vi "Remove Type Specialization Structure.vi"(8 "error in (no error)":errorcluster, 11 "VI Ref In":refnum<vi>) -> (0 "error out":errorcluster, 3 "VI Ref Out":refnum<vi>)   [LabVIEW 2020]
doc: "Removes the Type Specialization structure from the VI. The active case is first shown, then the structure removed to retain the correctly executable code."
uses:
  <vilib>/Utility/traverseref.llb/TRef TravTarget.ctl
  <vilib>/Utility/traverseref.llb/VI Scripting - Traverse.lvlib
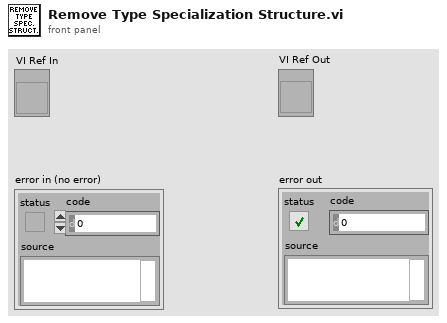
[diagram p1: front panel]
types:
  T1 = typedef "TRef TravTarget.ctl" = enum16{"FP", "BD", "Other"}
  T2 = enum32{"Conditional Disable Style", "Diagram Disable Style", "Type Specialization Style"}
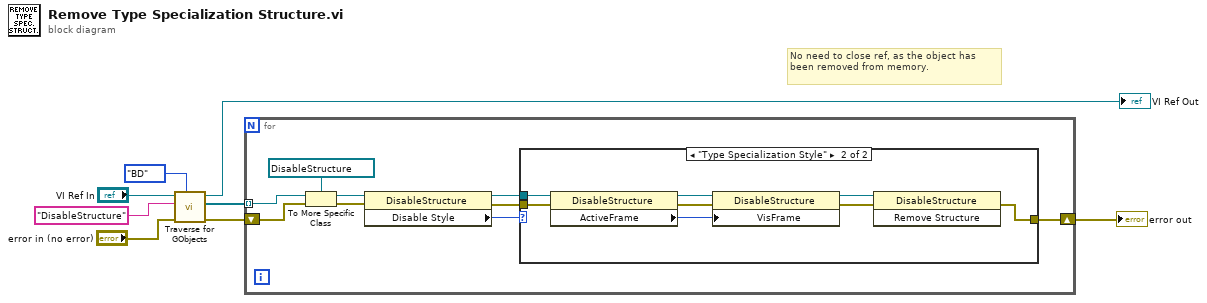
[diagram p0: block diagram]
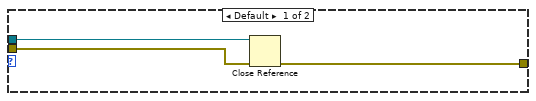
[diagram p2: hidden frame]
diagram:
  # "No need to close ref, as the object has been removed from memory."
  n1 = call <vilib>:"Traverse for GObjects.vi"("Traverse Target"=TRef_TravTarget."BD", "error in (no error)"="error in (no error)", "Class Name"="DisableStructure", "VI Refnum"="VI Ref In") -> ("error out"=w3:errorcluster, "References"=w5:refnum<vi>[], "dup VI Refnum"=→"VI Ref Out":refnum<vi>)  [unwired: 4 in, 1 out]
  n2 = for {
    tunnel: w5 -> [w16] mode=indexing
    shift-right: [w9] -> w2
    shift-left: w3 -> [w13]
    n3 = To More Specific Class(target class=refnum<vi> refnum ("reference"), reference=w16, error in=w13) -> (specific class reference=w15:refnum<vi>, error out=w12:errorcluster)
    n4 = property class="DisableStructure"(reference=w15, error in=w12) -> (reference out=w10:refnum<vi>, error out=w11:errorcluster, "Disable Style"=w14:T2)
    n5 = case shown="\"Type Specialization Style\"" w14 {
      tunnel: w11 -> [w19 w24]
      tunnel: w10 -> [w20 w25]
      tunnel: [w18 w21] -> w9
      frame Default {
        n6 = Close Reference(reference=w20, error in (no error)=w19) -> (error out=w18:errorcluster)
      }
      frame "Type Specialization Style" {
        n7 = property class="DisableStructure"(reference=w25, error in=w24) -> (reference out=w28:refnum<vi>, error out=w23:errorcluster, "ActiveFrame"=w27:i16)
        n8 = property class="DisableStructure"(reference=w28, error in=w23, "VisFrame"=w27) -> (reference out=w26:refnum<vi>, error out=w22:errorcluster)
        n9 = invoke class="DisableStructure" method="Remove Structure"(reference=w26, error in=w22) -> (error out=w21:errorcluster)  [unwired: 1 in, 2 out]
      }
    }
  }
  "error out" <- w2
